vi "AD7714 Wait on DRDY.vi"(10 "Channel":i16, 11 "I/O Cluster In":T1) -> (1 "Raw Response":bool[](array[boolean]), 2 "DRDY Iter":i32, 3 "I/O Cluster Out":T1)   [LabVIEW 2018, in "jmslib.lvlib"]
uses:
  jmslib.lvlib
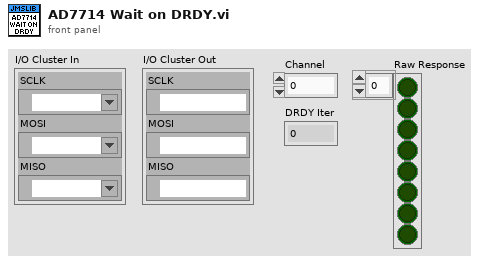
[diagram p1: front panel]
types:
  T1 = cluster{"SCLK":refnum<k21>, "MOSI":refnum<k21>, "MISO":refnum<k21>}
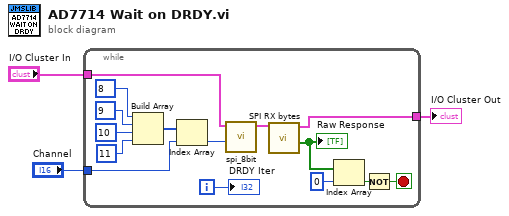
[diagram p0: block diagram]
diagram:
  n1 = while {
    tunnel: "Channel" -> [w14]
    tunnel: "I/O Cluster In" -> [w8]
    tunnel: [w4] -> w1
    i -> [w15]
    stop <- w17 stop-if-true
    n2 = Build Array(i8 8, i8 9, i8 10, i8 11) -> (w7:i8[])
    n3 = Index Array(array=w7, index=w14) -> (element=w9:i8)
    n4 = call "spi_8bit.vi"("Hex"=w9, "I/O Cluster In"=w8) -> ("I/O Cluster Out"=w5:T1)  [unwired: 9 in]
    n5 = call "SPI RX bytes.vi"("I/O Cluster In"=w5) -> ("Output Byte"=w6:bool[], "I/O Cluster Out"=w4:T1)  [unwired: 9 in]
    "Raw Response" <- w6
    n6 = Index Array(array=w6, index=0) -> (element=w16:bool)
    n7 = Not(x=w16) -> (.not. x?=w17:bool)
    "DRDY Iter" <- w15
  }
  "I/O Cluster Out" <- w1
